vi "HPF.vi"(6 "HPF enable":bool, 8 "error in (no error)":errorcluster, 11 "reference":refnum<k24>) -> (0 "error out":errorcluster, 3 "reference out":refnum<k24>)   [LabVIEW 2017]
uses:
  DLL/Modbus.dll
panel:
  in  "SlaveID":u8=1
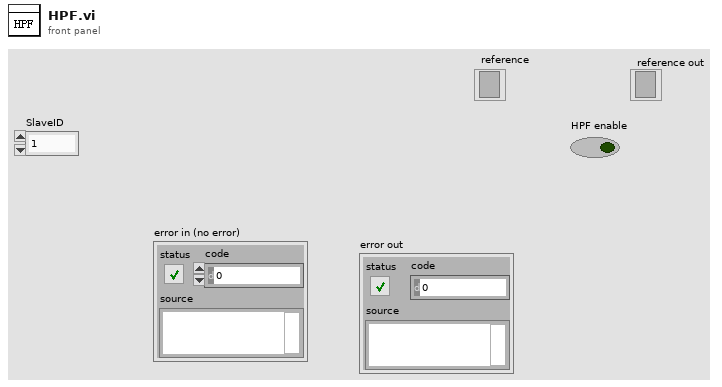
[diagram p1: front panel]
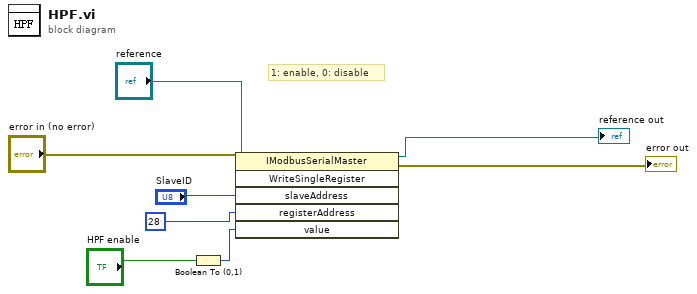
[diagram p0: block diagram]
diagram:
  # "1: enable, 0: disable"
  n1 = Boolean To (0,1)(Boolean="HPF enable") -> (0, 1=w2:i16)
  n2 = invoke class="IModbusSerialMaster" method="WriteSingleRegister"(reference="reference", error in="error in (no error)", "slaveAddress"="SlaveID", "registerAddress"=u16 28 ("numberOfPoints"), "value"=w2) -> (reference out=→"reference out":refnum<k24>, error out=→"error out":errorcluster)  [unwired: 1 in, 4 out]
